vi "GetRawWaveform.vi"(8 "error in":errorcluster {"code" format="%.0x"}, 11 "VISA Resource Name":refnum<visa-resource-name>) -> (0 "error out":errorcluster {"code" format="%.0x"}, 1 "Waveform Array":u32[](array[numeric]), 2 "Number of Points":u32, 3 "VISA Resource Name Out":refnum<visa-resource-name>, 4 "Size of Point":u32)   [LabVIEW 2011, in "Agilent 546XX Series.lvlib"]
uses:
  Agilent 546XX Series.lvlib
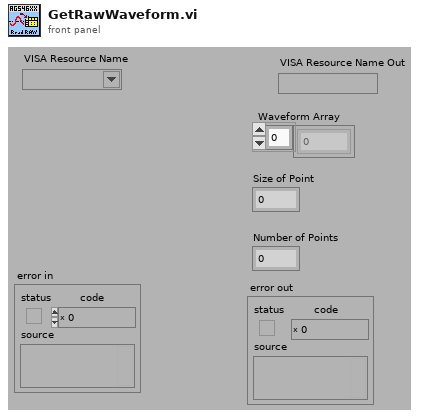
[diagram p1: front panel]
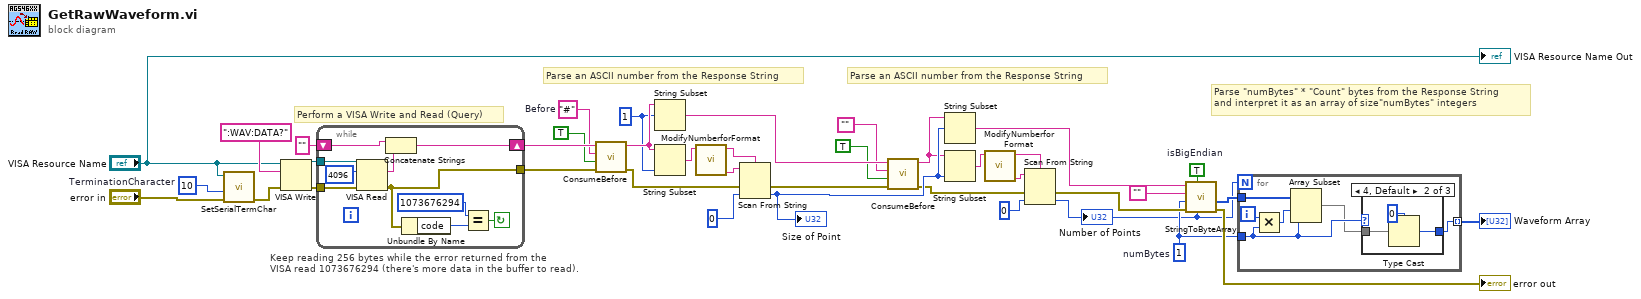
[diagram p0: block diagram]
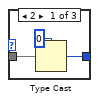
[diagram p2: hidden frame]
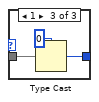
[diagram p3: hidden frame]
diagram:
  w17 = TRUE  # isBigEndian
  w11 = u32 1  # numBytes
  w25 = u32 1 ("StringLength")
  w28 = "#"  # Before
  w33 = u8 10  # TerminationCharacter
  # "Parse \"numBytes\" * \"Count\" bytes from the Response String\nand interpret it as an array of size\"numBytes\" integers"
  # "Parse an ASCII number from the Response String"
  # "Parse an ASCII number from the Response String"
  # "Perform a VISA Write and Read (Query)"
  # "Keep reading 256 bytes while the error returned from the\nVISA read 1073676294 (there's more data in the buffer to read)."
  n1 = call "SetSerialTermChar.vi"("error IO"="error in", "termination char\n(0xA = '\\n' = LF)"=w33, "VISA resource name"="VISA Resource Name") -> ("error IO 2"=w32:errorcluster)  [unwired: 8 in]
  n2 = VISA Write(VISA resource name="VISA Resource Name", write buffer=":WAV:DATA?" ("Command"), error in (no error)=w32) -> (VISA resource name out=w39:refnum<visa-resource-name>, error out=w37:errorcluster)  [unwired: 1 out]
  n3 = while {
    tunnel: w39 -> [w46]
    shift-right: [w44] -> w38
    shift-left: "" -> [w40]
    tunnel: w37 -> [w43]
    tunnel: [w41] -> w36
    stop <- w42 continue-if-true
    n4 = VISA Read(VISA resource name=w46, byte count=u32 4096 ("byte count (0)"), error in (no error)=w43) -> (read buffer=w45:string, error out=w41:errorcluster)  [unwired: 2 out]
    n5 = Concatenate Strings(w40, w45) -> (w44:string)
    n6 = Unbundle By Name(w41) -> ("code"=w48:i32)
    n7 = Equal?(x=1073676294, y=w48) -> (x = y?=w42:bool)
  }
  n8 = call "ConsumeBefore.vi"("error in"=w36, "ASCII"=TRUE, "Before"=w28, "Response String In"=w38) -> ("error out"=w23:errorcluster, "Response String Out"=w26:string)  [unwired: 6 in]
  n9 = String Subset(string=w26, offset (0)=w25) -> (substring=w24:string)  [unwired: 1 in]
  n10 = String Subset(string=w26, length (rest)=w25) -> (substring=w6:string)  [unwired: 1 in]
  n11 = call "ModifyNumberforFormat.vi"("String to modify"=w6) -> ("Modified string"=w5:string, "Format"=w4:string)  [unwired: 9 in]
  n12 = Scan From String(format string=w4, input string=w5, error in=w23, default 1=u32 0 ("Default Value 1")) -> (error out=w27:errorcluster, output 1=w29:u32)  [unwired: 1 in, 2 out]
  "Size of Point" <- w29
  n13 = call "ConsumeBefore.vi"("error in"=w27, "ASCII"=TRUE, "Before"="", "Response String In"=w24) -> ("error out"=w18:errorcluster, "Response String Out"=w19:string)  [unwired: 6 in]
  n14 = String Subset(string=w19, offset (0)=w29) -> (substring=w8:string)  [unwired: 1 in]
  n15 = String Subset(string=w19, length (rest)=w29) -> (substring=w3:string)  [unwired: 1 in]
  n16 = call "ModifyNumberforFormat.vi"("String to modify"=w3) -> ("Modified string"=w1:string, "Format"=w2:string)  [unwired: 9 in]
  n17 = Scan From String(format string=w2, input string=w1, error in=w18, default 1=u32 0 ("Default Value 1")) -> (error out=w20:errorcluster, output 1=w10:u32)  [unwired: 1 in, 2 out]
  "Number of Points" <- w10
  n18 = call "StringToByteArray.vi"("count"=w10, "isBigEndian"=w17, "error in"=w20, "numBytes"=w11, "Before"="", "ResponseStringIn (01 23 45 67 89 AB CD EF FF EE)"=w8) -> ("errorout"=→"error out":errorcluster, "Array"=w16:u8[])  [unwired: 3 in, 1 out]
  n19 = for {
    N: w10 -> [_]
    tunnel: w11 -> [w52]
    tunnel: [w50] -> w12 mode=indexing
    tunnel: w16 -> [w55]
    i -> [w53]
    n20 = Multiply(x=w53, y=w52) -> (x*y=w54:u32)
    n21 = Array Subset(array=w55, index=w54, length=w52) -> (w51:u8[])
    n22 = case shown="4, Default" w52 {
      tunnel: w51 -> [w57 w61 w64]
      tunnel: [w58 w60 w63] -> w50
      frame 2 {
        n23 = Type Cast(type=u16 0, x=w57) -> (*(type *) &x=w58:u16)
      }
      frame 4, Default {
        n24 = Type Cast(type=u32 0, x=w61) -> (*(type *) &x=w60:u32)
      }
      frame 1 {
        n25 = Type Cast(type=u8 0, x=w64) -> (*(type *) &x=w63:u8)
      }
    }
  }
  "Waveform Array" <- w12
  "VISA Resource Name Out" <- "VISA Resource Name"
